vi "SHaredVariableSaver.vi"(0 "shared variable refnum in":refnum<k21>, 1 "cmd":enum16{"read from file", "write to file"}(ring), 2 "dir":path, 11 "error in (no error)":errorcluster) -> (15 "error out":errorcluster)   [LabVIEW 2019]
uses:
  ConfigJSON_class/ConfigJSON.lvclass
  ConfigJSON_class/ConfigJSON.lvclass/ConfigJSON.ctl
  fcae2cab-1ade-4f92-8207-1c3d14f200db.vi
  <vilib>/Utility/error.llb/Clear Errors.vi
  <resource>/objmgr/ni.var.rc
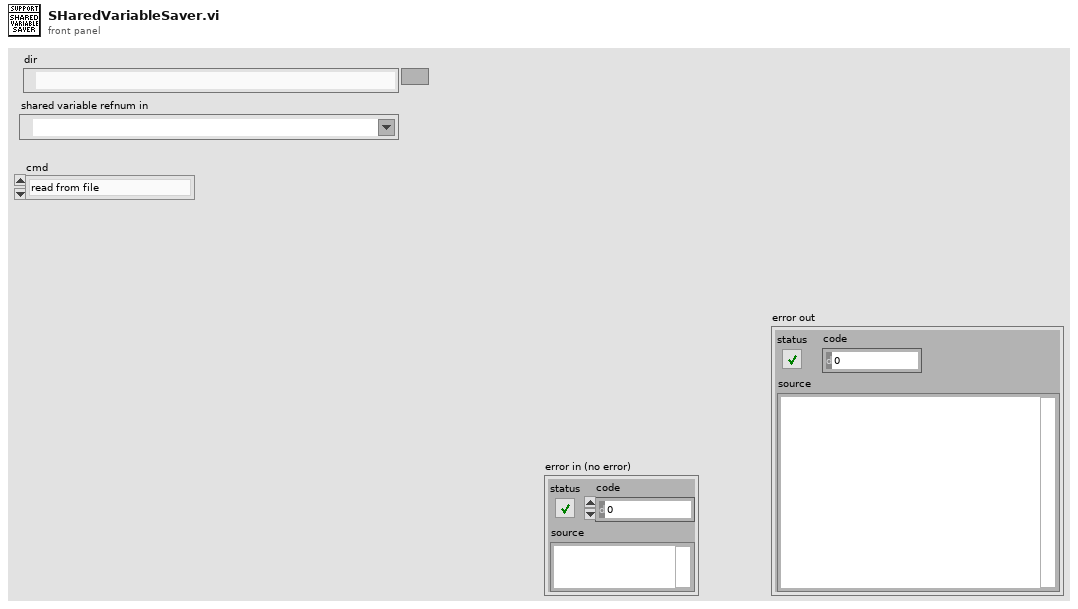
[diagram p1: front panel]
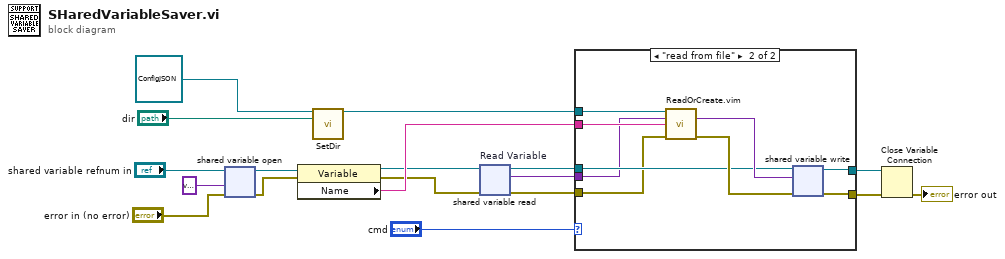
[diagram p0: block diagram]
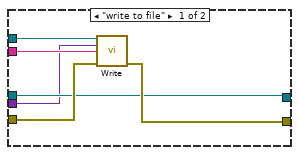
[diagram p2: hidden frame]
diagram:
  n1 = shared-variable-open("shared variable refnum in", "error in (no error)", variant) -> (w10:refnum<k21>, w9:errorcluster)  [unwired: 1 in]
  n2 = property class="Variable"(reference=w10, error in=w9) -> (reference out=w6:refnum<k21>, error out=w5:errorcluster, "Name"=w8:string)
  n3 = call "SetDir.vi"("reference in"=refnum<class "ConfigJSON.lvclass"> refnum, "Config Dir"="dir") -> ("JSON"=w12:refnum<class "ConfigJSON.lvclass">)  [unwired: 13 in]
  n4 = shared-variable-read "Read Variable"(w6, w5) -> (w3:refnum<k21>, w4:errorcluster, w2:variant)  [unwired: 1 out]
  n5 = case shown="\"read from file\"" "cmd" {
    tunnel: [w24 w31] -> w13
    tunnel: w12 -> [w23 w33]
    tunnel: [w21 w30] -> w11
    tunnel: w4 -> [w22 w26]
    tunnel: w3 -> [w21 w27]
    tunnel: w8 -> [w20 w32]
    tunnel: w2 -> [w19 w25]
    frame "write to file" {
      n6 = call-dynamic "Write.vi"("reference in"=w23, "Data"=w19, "Name"=w20, "error in (no error)"=w22) -> ("error out"=w24:errorcluster)  [unwired: 8 in, 3 out]
    }
    frame "read from file" {
      n7 = call "ReadOrCreate.vim"("reference in"=w33, "Type and Defaults"=w25, "Name"=w32, "error in (no error)"=w26) -> ("Data"=w28:variant, "error out"=w29:errorcluster)  [unwired: 7 in, 3 out]
      n8 = shared-variable-write(w27, w29, w28) -> (w30:refnum<k21>, w31:errorcluster)
    }
  }
  n9 = Close Variable Connection(8:w13, 11:w11) -> (0:→"error out":errorcluster)
